vi "Get Destination Name.vi"(8 "error in (no error)":errorcluster, 10 "Default Destinations":T1, 11 "SDIST in":refnum<class "NI_AB_API_SDIST.lvclass">) -> (0 "error out":errorcluster, 2 "Destination Name":string, 3 "SDIST out":refnum<class "NI_AB_API_SDIST.lvclass">)   [LabVIEW 2020, in "NI_AB_API_SDIST.lvclass"]
uses:
  <vilib>/AppBuilder/AB_API/SDIST/NI_AB_API_SDIST.lvclass
  <vilib>/AppBuilder/AB_API/common/AB_API Default Destinations.ctl
  <vilib>/AppBuilder/AB_API/Build/NI_AB_API_Build.lvclass
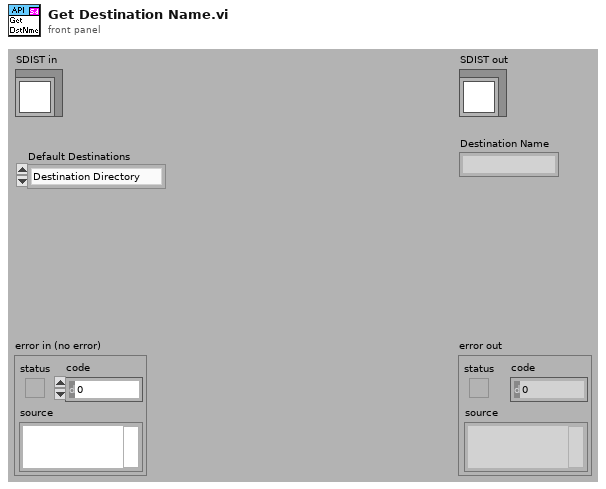
[diagram p1: front panel]
types:
  T1 = typedef "AB_API Default Destinations.ctl" = enum16{"Destination Directory", "Support Directory"}
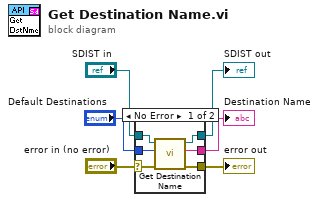
[diagram p0: block diagram]
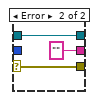
[diagram p2: hidden frame]
diagram:
  n1 = case shown="No Error" "error in (no error)" {
    selector: "error in (no error)" -> [w12 w15]
    tunnel: [w8 w15] -> w5
    tunnel: [w10 w14] -> w3
    tunnel: "SDIST in" -> [w11 w14]
    tunnel: "Default Destinations" -> [w7 _]
    tunnel: [w9 "" ("Destination Name")] -> w2
    frame No Error {
      n2 = call-parent "Get Destination Name.vi"("error in (no error)"=w12, "Default Destinations"=w7, "NI_AB_API_Build in"=w11) -> ("error out"=w8:errorcluster, "Destination Name"=w9:string, "NI_AB_API_Build out"=w10:refnum<class "NI_AB_API_SDIST.lvclass">)  [unwired: 6 in]
    }
    frame Error {
    }
  }
  "error out" <- w5
  "SDIST out" <- w3
  "Destination Name" <- w2
